vi "DDG Check Multi Module Global Channels.vi"(0 "Global Channel In":refnum<k21>, 11 "error in (no error)":errorcluster) -> (4 "Global Channel Out":refnum<k21>, 15 "error out":errorcluster)   [LabVIEW 2021, in "DAQ_Dynamic Digital Pattern Generation.lvlib"]
doc: "checks for the presence of multiple module global channels and throws the error if identified"
uses:
  DAQ_Dynamic Digital Pattern Generation.lvlib
  <vilib>/Utility/error.llb/Error Cluster From Error Code.vi
  <vilib>/ErrorRing/Error Ring.xnode
  <resource>/objmgr/daqmx.rc
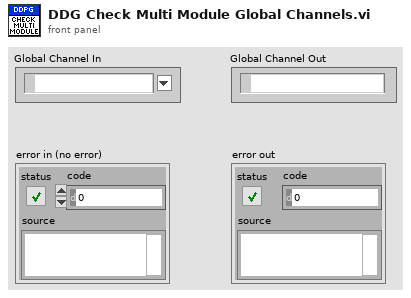
[diagram p1: front panel]
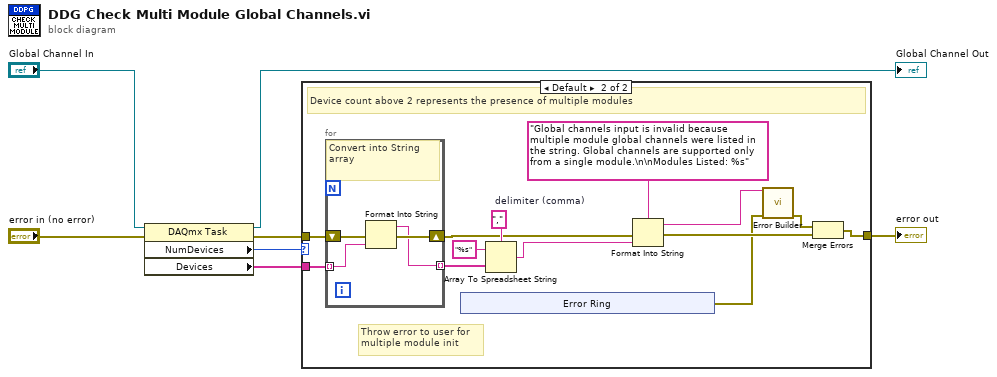
[diagram p0: block diagram]
diagram:
  n1 = property class="DAQmx Task"(reference="Global Channel In", error in="error in (no error)") -> (reference out=→"Global Channel Out":refnum<k21>, error out=w5:errorcluster, "NumDevices"=w4:u32, "Devices"=w2:tag[])
  n2 = case shown="Default" w4 {
    tunnel: w5 -> [w8 w20]
    tunnel: w2 -> [_ w21]
    tunnel: [w8 w9] -> w1
    frame 1, 2 {
      # "Only 1 module is present other than TS backpane"
    }
    frame Default {
      w18 = ","  # delimiter (comma)
      # "Throw error to user for \nmultiple module init"
      # "Device count above 2 represents the presence of multiple modules"
      n3 = for {
        tunnel: w21 -> [w28] mode=indexing
        shift-right: [w27] -> w11
        shift-left: w20 -> [w29]
        tunnel: [w26] -> w19 mode=indexing
        # "Convert into String array"
        n4 = Format Into String(error in=w29, w28) -> (resulting string=w26:string, error out=w27:errorcluster)  [unwired: 2 in]
      }
      n5 = xnode "Error Ring"() -> ("error out"=w13:errorcluster)
      n6 = Array To Spreadsheet String(delimiter (Tab)=w18, array=w19, 3:"%s" ("format string")) -> (spreadsheet string=w10:string)
      n7 = Format Into String(format string="Global channels input is invalid because multiple module global channels were listed in the string. Global channels are supported only from a single module.\n\nModules Listed: %s" ("error message (\"\")"), error in=w11, w10) -> (resulting string=w16:string, error out=w14:errorcluster)  [unwired: 1 in]
      n8 = call "Error Builder.vi"("Error String"=w16, "Error In"=w13) -> ("Error Out"=w15:errorcluster)  [unwired: 13 in]
      n9 = Merge Errors(w15, w14) -> (w9:errorcluster)
    }
  }
  "error out" <- w1
